vi "UserVars-Expression to Vector.vi"(7 "Expr":string, 11 "error in (no error)":errorcluster, 13 "Nrand":i32=1) -> (8 "Values":dbl[](array[numeric]), 15 "error out":errorcluster)   [LabVIEW 2020]
uses:
  <vilib>/gmath/NI_Gmath.lvlib
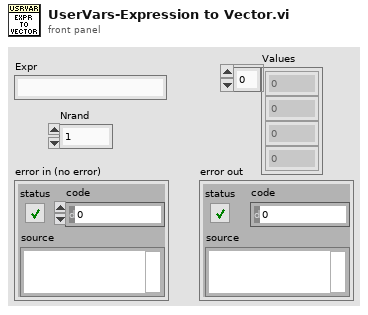
[diagram p1: front panel]
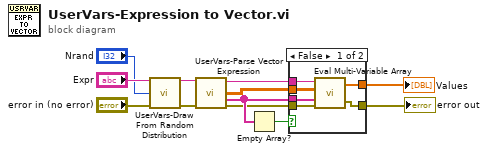
[diagram p0: block diagram]
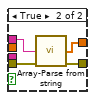
[diagram p2: hidden frame]
diagram:
  n1 = call "UserVars-Draw From Random Distribution.vi"("Expr in"="Expr", "Nrand"="Nrand", "error in (no error)"="error in (no error)") -> ("Expr out"=w5:string, "error out"=w4:errorcluster)  [unwired: 11 in]
  n2 = call "UserVars-Parse Vector Expression.vi"("Expression In"=w5, "error in (no error)"=w4) -> ("Expression Out"=w6:string, "values"=w7:dbl[][], "variables"=w11:string[], "error out"=w8:errorcluster)  [unwired: 10 in]
  n3 = Empty Array?(array=w11) -> (empty?=w12:bool)
  n4 = case shown="False" w12 {
    tunnel: w6 -> [w18 w21]
    tunnel: w7 -> [w17 _]
    tunnel: w11 -> [w16 _]
    tunnel: w8 -> [w15 w19]
    tunnel: [w14 w22] -> w9
    tunnel: [w13 w20] -> w10
    frame False {
      n5 = call <vilib>:"Eval Multi-Variable Array.vi"("error in (no error)"=w15, "Variables"=w16, "X Values"=w17, "formula"=w18) -> ("error out"=w14:errorcluster, "Y Values"=w13:dbl[])
    }
    frame True {
      n6 = call "Array-Parse from string.vi"("String"=w21, "error in (no error)"=w19) -> ("Array"=w20:dbl[], "error out"=w22:errorcluster)  [unwired: 12 in]
    }
  }
  "error out" <- w9
  "Values" <- w10
